vi "Select Device.vi"(2 "error in (no error)":errorcluster, 3 "Device":i32) -> (0 "error out":errorcluster, 1 "function return":i32)   [LabVIEW 2014, in "MCM3000.lvlib"]
doc: "long SelectDevice(const long Device);"
uses:
  MCM3000.lvlib
  ThorMCM3000.dll
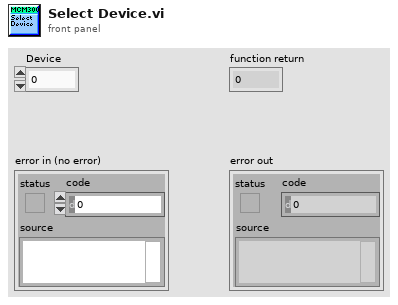
[diagram p1: front panel]
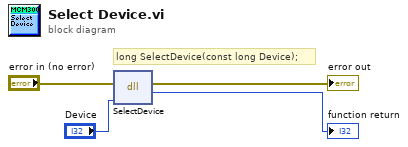
[diagram p0: block diagram]
diagram:
  # "long SelectDevice(const long Device);"
  n1 = dll-call lib="C:/TIS_CalebVS2012/TIS_Development/Hardware/SDKs/MCM3000_SDK/LabVIEW/inc/ThorMCM3000.*" fn="SelectDevice"(error in="error in (no error)", "Device"="Device") -> (error out=→"error out":errorcluster, →"function return":i32)  [unwired: 3 in, 1 out]
